vi "EXECUTION_UI.vi"(8 "error in (no error)":errorcluster, 11 "Execution in":refnum<data-value>) -> (0 "error out":errorcluster, 3 "Execution out":refnum<data-value>)   [LabVIEW 2015, in "Execution.lvclass"]
uses:
  Execution.lvclass
  EXECUTION_UI_MSG.ctl
  EXECUTION_CTRL_MSG.ctl
  <vilib>/Utility/miscctls.llb/LVRectTypeDef.ctl
  <vilib>/Utility/miscctls.llb/LVPointTypeDef.ctl
  <vilib>/Utility/miscctls.llb/LVRowAndColumnTypeDef.ctl
  DUT_INFO_TYPEDEF.ctl
  EXECUTION_RESULT_TYPEDEF.ctl
  EXECUTION_STATUS.ctl
  BACKGROUND_CONTROL_MSG_TYPEDEF.ctl
  Step/STEP_STATUS.ctl
  STEP_END_DATA_TYPEDEF.ctl
  <vilib>/Utility/miscctls.llb/LVRowAndColumnUnsignedTypeDef.ctl
  Send UI Message.vi
  Send Control Message.vi
  Project.lvclass
  Step.lvclass
panel:
  out "STOP_FLAG":bool
  out "TEST_TIME":string
  in  "MENU_BTN":bool
  in  "CTRL_BTN":bool
  out "PROGRASS_BAR":u8(slide) scale=0.0..100.0
  out "STATUS":string
  out "SN":string
  out "TEST_TABLE":string[][](table)
  out "Msg":string
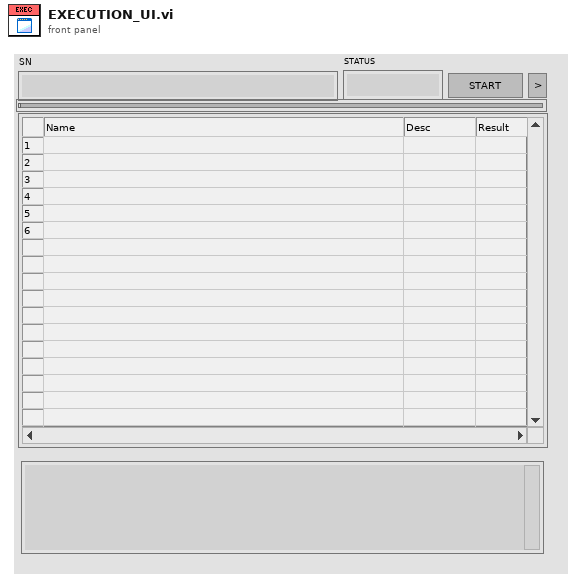
[diagram p1: front panel]
types:
  T1 = typedef "Execution.lvclass/EXECUTION_UI_MSG.ctl" = enum16{"EXECUTION_STATUS", "INIT_UI", "DUT_UPDATE", "BOTTOM_PANEL_UPDATE", "TOP_PANEL_UPDATE", "STEP_START", "STEP_END", "DISPLAY_RESULT", "APPLICATION_END"}
  T2 = typedef "LVRectTypeDef.ctl" = cluster{"Left":i16, "Top":i16, "Right":i16, "Bottom":i16}
  T3 = typedef "LVPointTypeDef.ctl" = cluster{"Horizontal":i16, "Vertical":i16}
  T4 = typedef "LVRowAndColumnTypeDef.ctl" = cluster{"Row":i32, "Column":i32}
  T5 = typedef "Execution.lvclass/DUT_INFO_TYPEDEF.ctl" = cluster{"SN":string, "Model":string, "PartNumber":string, "Revision":string, "Software":string, "Hardware":string}
  T6 = typedef "Execution.lvclass/EXECUTION_RESULT_TYPEDEF.ctl" = enum16{"Unknow", "Terminated", "Passed", "Failed", "Error"}
  T7 = typedef "Execution.lvclass/EXECUTION_STATUS.ctl" = enum16{"Initializing ", "Disable", "Ready", "Running", "Finished"}
  T8 = enum8{"Enabled", "Disabled", "Disabled and Grayed Out"}
  T9 = typedef "Execution.lvclass/BACKGROUND_CONTROL_MSG_TYPEDEF.ctl" = cluster{"Target":string, "Msg":string, "Data":variant}
  T10 = typedef "LVRowAndColumnUnsignedTypeDef.ctl" = cluster{"Row":u32, "Column":u32}
  T11 = typedef "Execution.lvclass/STEP_END_DATA_TYPEDEF.ctl" = cluster{"Index":i32, "Result":T12, "Duration":dbl, "Value":string, "Low Limit":string, "Upper Limit":string}
  T12 = typedef "Step.lvclass/STEP_STATUS.ctl" = enum16{"Skipped", "Done", "Passed", "Failed", "Error"}
  T13 = typedef "Execution.lvclass/EXECUTION_CTRL_MSG.ctl" = enum16{"EXECUTION_START", "EXECUTION_END", "EXECUTION_LOOP", "APPLICATION_STOP"}
  T14 = typedef "Execution.lvclass/EXECUTION_UI_QUEUE_DATA.ctl" = cluster{"Msg":T1, "Data":variant}
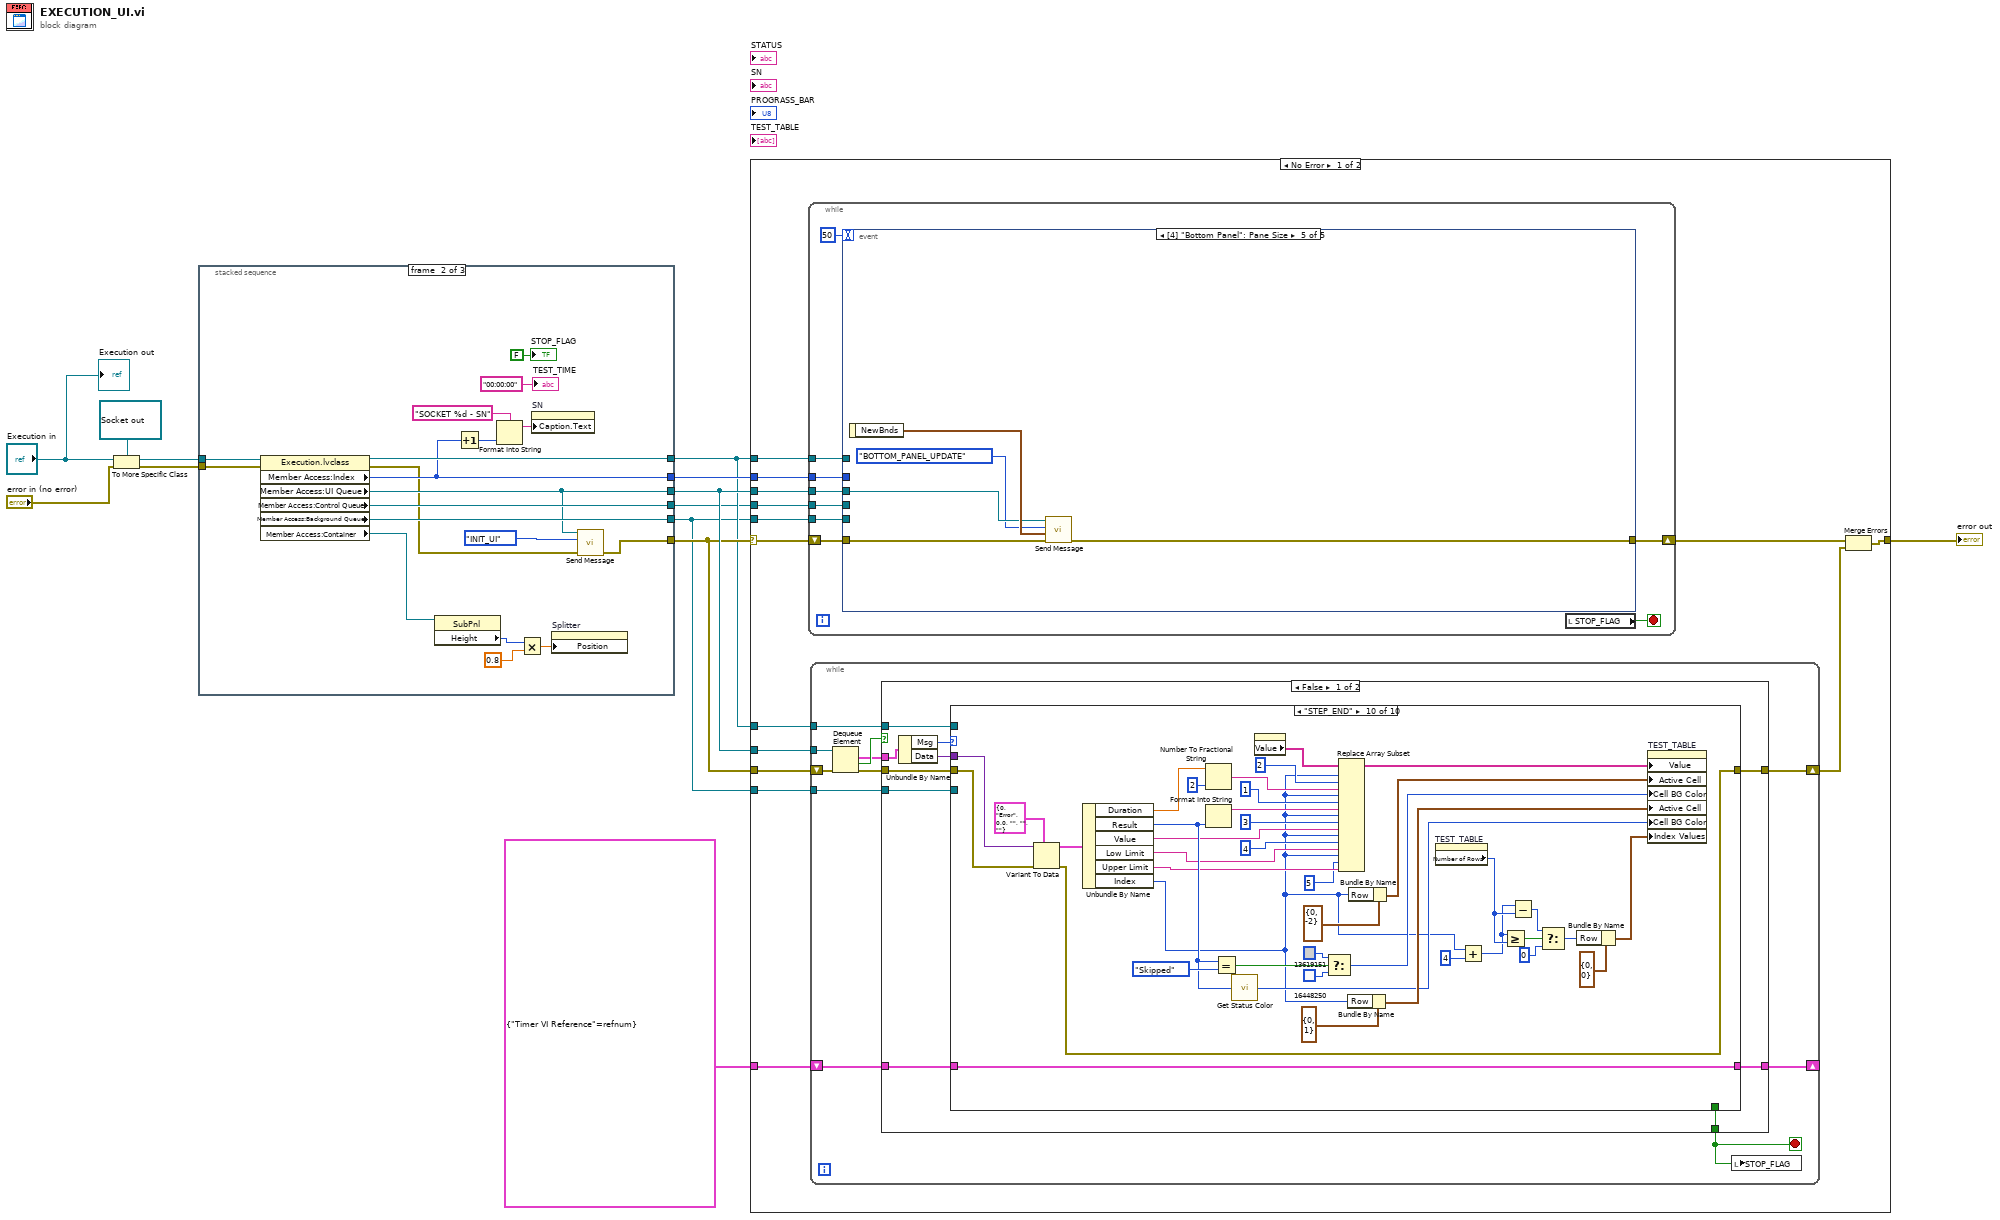
[diagram p0: block diagram]
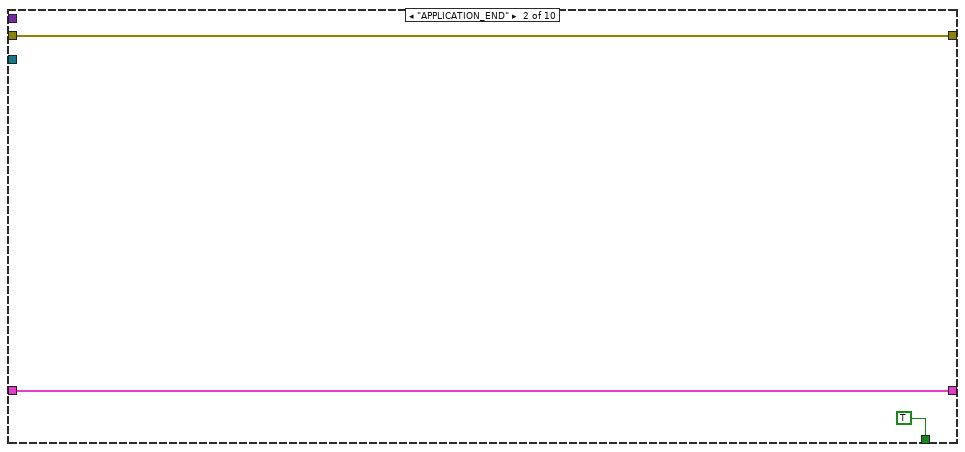
[diagram p5: hidden frame]
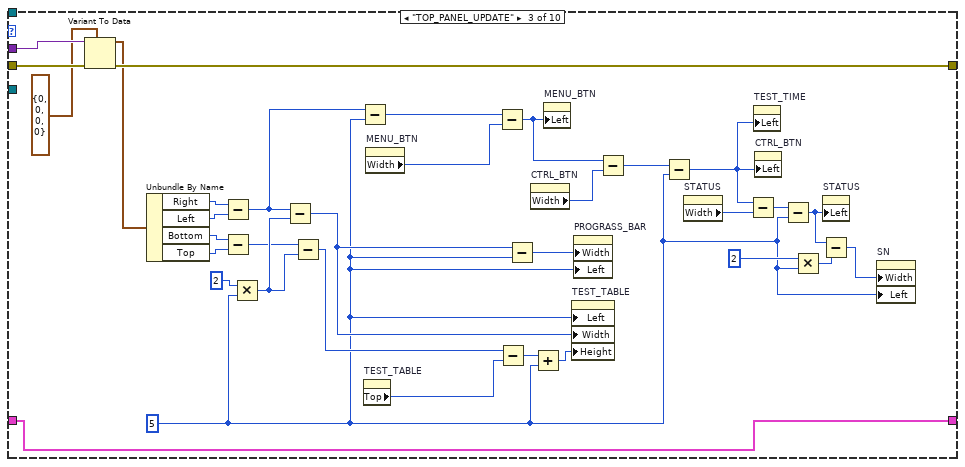
[diagram p6: hidden frame]
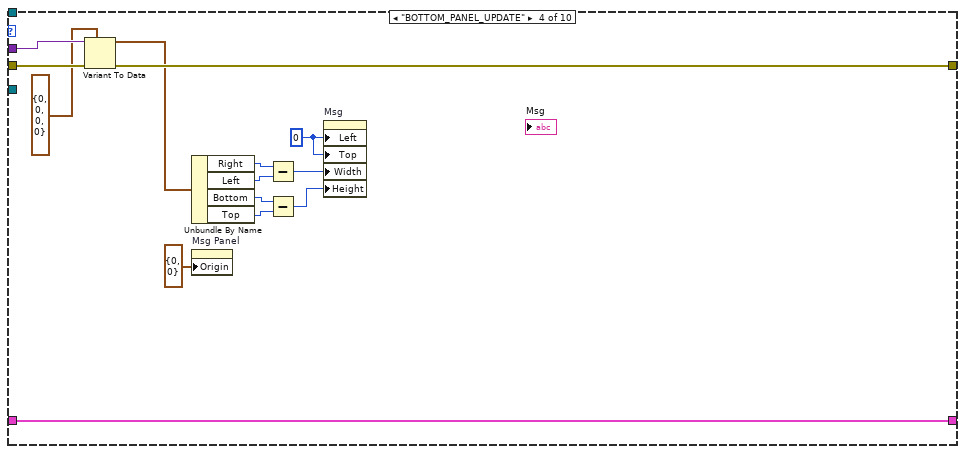
[diagram p7: hidden frame]
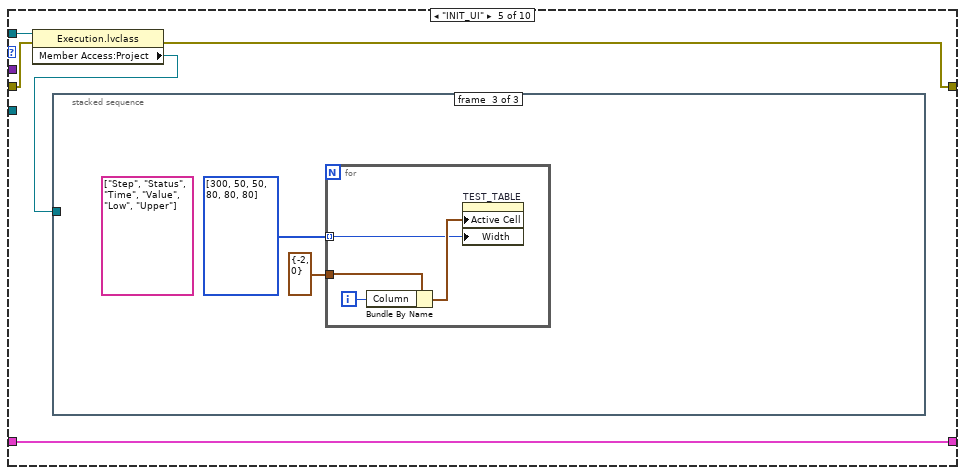
[diagram p8: hidden frame]
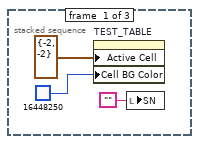
[diagram p9: hidden frame]
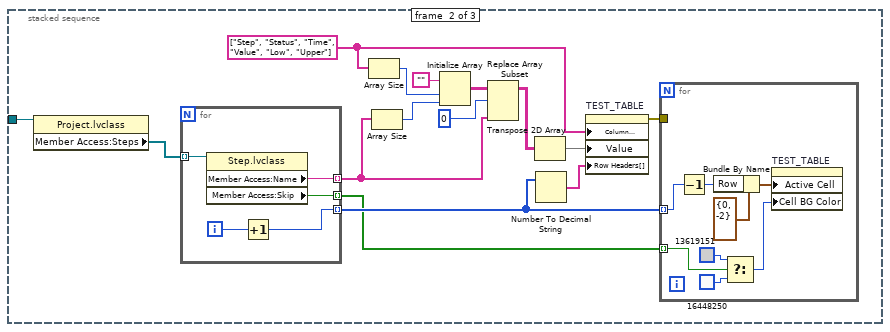
[diagram p10: hidden frame]
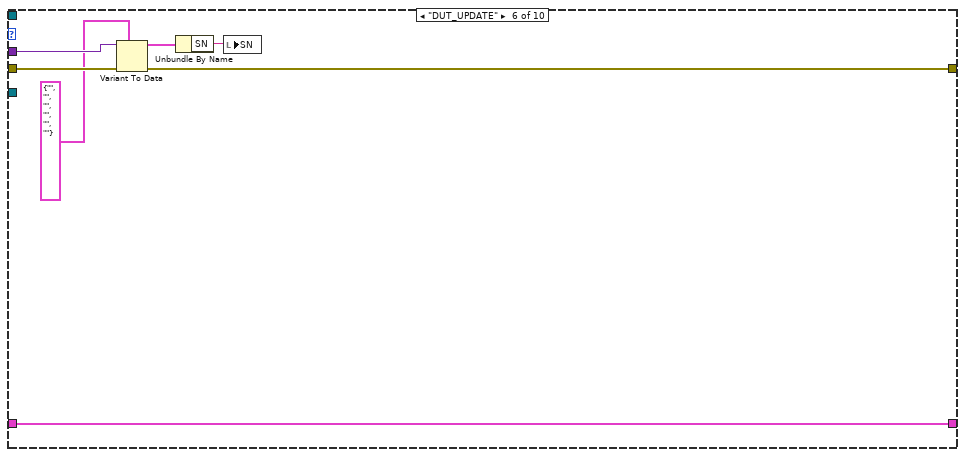
[diagram p11: hidden frame]
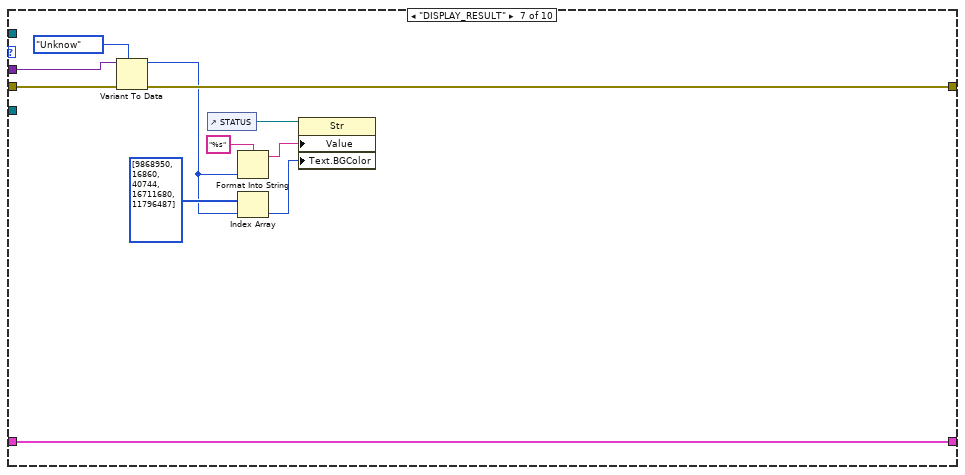
[diagram p12: hidden frame]
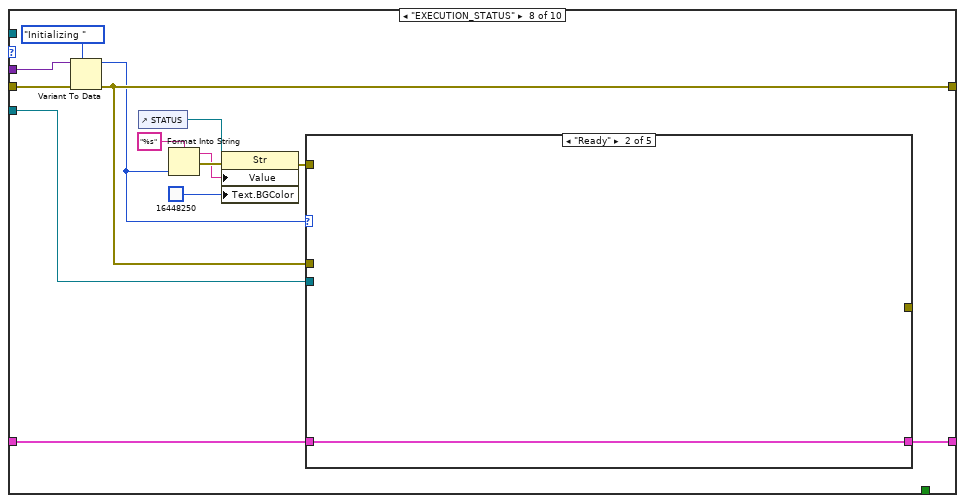
[diagram p13: hidden frame]
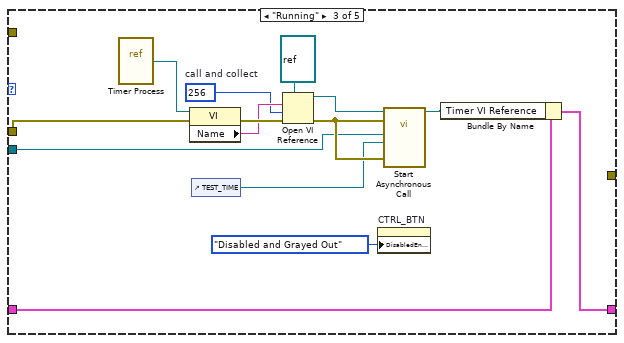
[diagram p15: hidden frame]
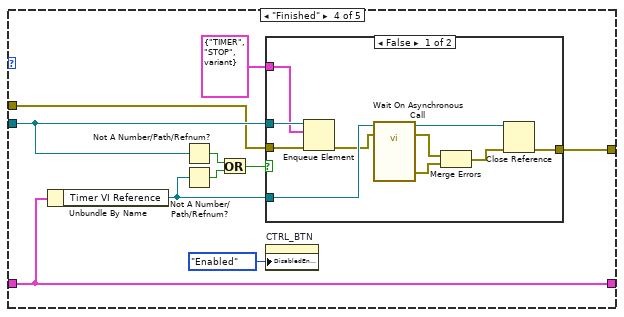
[diagram p16: hidden frame]
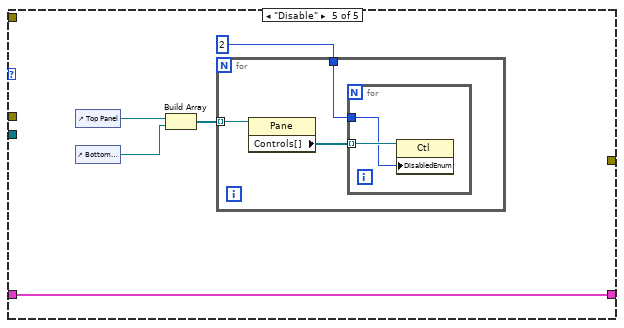
[diagram p18: hidden frame]
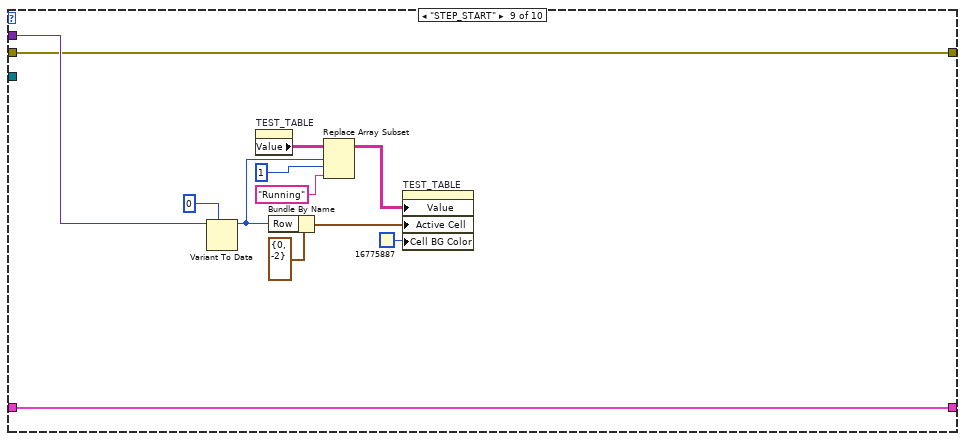
[diagram p19: hidden frame]
diagram:
  n1 = To More Specific Class(target class=refnum<data-value> refnum ("reference out"), reference="Execution in", error in="error in (no error)") -> (specific class reference=w3:refnum<data-value>, error out=w1:errorcluster)
  n2 = stacked-sequence {
    tunnel: [_ w27 _] -> w12
    tunnel: [_ w17 _] -> w11
    tunnel: [_ w14 _] -> w10
    tunnel: [_ w32 _] -> w8
    tunnel: [_ w21 _] -> w7
    tunnel: [_ w20 _] -> w6
    tunnel: w3 -> [_ w19 _]
    tunnel: w1 -> [_ w18 _]
    frame #0 {
    }
    frame #1 {
      n3 = property class="Execution.lvclass"(reference=w19, error in=w18) -> (reference out=w32:refnum<data-value>, error out=w15:errorcluster, "Member Access:Index"=w27:u8, "Member Access:UI Queue"=w17:refnum<queue>, "Member Access:Control Queue"=w20:refnum<queue>, "Member Access:Background Queue"=w21:refnum<queue>, "Member Access:Container"=w22:refnum<vi>)
      n4 = property class="SubPnl"(reference=w22) -> ("Height"=w31:u32)  [unwired: 1 in, 2 out]
      n5 = Increment(x=w27) -> (x+1=w25:u8)
      n6 = Format Into String(format string="SOCKET %d - SN", w25) -> (resulting string=w24:string)  [unwired: 2 in, 1 out]
      n7 = Multiply(x=w31, y=0.8) -> (x*y=w30:dbl)
      n8 = property on="SN" class="Str"("Caption.Text"=w24) -> ()  [unwired: 2 in, 2 out]
      n9 = property on="Splitter" class="Splitter"("Position"=w30) -> ()  [unwired: 2 in, 2 out]
      n10 = call-poly "Send Message.vi"("error in (no error)"=w15, "Msg"=EXECUTION_UI_MSG."INIT_UI", "UI Queue"=w17) -> ("error out"=w14:errorcluster)  [unwired: 8 in]
      "TEST_TIME" <- "00:00:00" ("String")
      "STOP_FLAG" <- FALSE ("STOP_FLAG")
    }
    frame #2 {
    }
  }
  n11 = case shown="No Error" w10 {
    selector: w10 -> [w46 w319]
    tunnel: [w38 w319] -> w13
    tunnel: w11 -> [w45 _]
    tunnel: w12 -> [w44 _]
    tunnel: w8 -> [w43 _]
    tunnel: w11 -> [w42 _]
    tunnel: w10 -> [w41 _]
    tunnel: w7 -> [w37 _]
    tunnel: cluster{"Timer VI Reference":refnum<vi>} {"Timer VI Reference"=refnum} -> [w36 _]
    tunnel: w8 -> [w35 _]
    tunnel: w7 -> [w34 _]
    tunnel: w6 -> [w33 _]
    frame No Error {
      n12 = while {
        tunnel: w45 -> [w300]
        tunnel: w44 -> [w299]
        shift-right: [w302] -> w40
        shift-left: w46 -> [w303]
        tunnel: w43 -> [w298]
        tunnel: w34 -> [w296]
        tunnel: w33 -> [w295]
        stop <- w297 stop-if-true
        n13 = event shown="[4] \"Bottom Panel\": Pane Size" {
          selector: _ -> [_ _ _ _ _]
          dyn-events: _ -> [_ _ _ _ _]
          timeout: 50 -> [_ _ _ _ _]
          tunnel: w303 -> [w304 w308 _ w313 w315]
          tunnel: [w304 w307 _ w309 w314] -> w302
          tunnel: w300 -> [_ _ _ w312 w317]
          tunnel: w299 -> [_ _ _ _ _]
          tunnel: w298 -> [_ _ _ _ _]
          tunnel: w296 -> [_ _ _ _ _]
          tunnel: w295 -> [_ w306 _ _ _]
          event Timeout {
            n14 = event-data() -> ()  [unwired: 1 in, 3 out]
          }
          event "CTRL_BTN": Value Change {
            n15 = event-data() -> ()  [unwired: 1 in, 6 out]
            n16 = call-poly "Send Message.vi"("error in (no error)"=w308, "Msg"=EXECUTION_CTRL_MSG."EXECUTION_START", "Control Queue"=w306) -> ("error out"=w307:errorcluster)  [unwired: 8 in]
          }
          event "MENU_BTN": Value Change {
            n17 = event-data() -> ()  [unwired: 1 in, 6 out]
          }
          event Pane Size {
            n18 = event-data() -> ("NewBnds"=w310:T2)  [unwired: 1 in]
            n19 = call-poly "Send Message.vi"("error in (no error)"=w313, "Data"=w310, "Msg"=EXECUTION_UI_MSG."TOP_PANEL_UPDATE", "UI Queue"=w312) -> ("error out"=w309:errorcluster)  [unwired: 7 in]
          }
          event Pane Size {
            n20 = event-data() -> ("NewBnds"=w318:T2)  [unwired: 1 in]
            n21 = call-poly "Send Message.vi"("error in (no error)"=w315, "Data"=w318, "Msg"=EXECUTION_UI_MSG."BOTTOM_PANEL_UPDATE", "UI Queue"=w317) -> ("error out"=w314:errorcluster)  [unwired: 7 in]
          }
        }
        n22 = local read "STOP_FLAG"() -> (w297:bool)
      }
      n23 = while {
        tunnel: w42 -> [w57]
        shift-right: [w52] -> w39
        shift-left: w41 -> [w56]
        tunnel: w37 -> [w49]
        shift-right: [w48] -> _
        shift-left: w36 -> [w50]
        tunnel: w35 -> [w47]
        stop <- w51 stop-if-true
        n24 = Dequeue Element(queue=w57, error in (no error)=w56) -> (element=w54:T14, timed out?=w55:bool, error out=w53:errorcluster)  [unwired: 1 in, 1 out]
        n25 = case shown="False" w55 {
          tunnel: w53 -> [w64 w294]
          tunnel: w54 -> [w65 _]
          tunnel: [w67 w294] -> w52
          tunnel: [w66 _] -> w51
          tunnel: w50 -> [w61 w293]
          tunnel: w49 -> [w60 _]
          tunnel: [w59 w293] -> w48
          tunnel: w47 -> [w58 _]
          frame False {
            n26 = Unbundle By Name(w65) -> ("Msg"=w63:T1, "Data"=w62:variant)
            n27 = case shown="\"STEP_END\"" w63 {
              tunnel: w64 -> [w69 w72 w78 w118 w121 w167 w178 w193 w247 w270]
              tunnel: [w69 w72 w77 w117 w120 w163 w177 w189 w247 w269] -> w67
              tunnel: [_ TRUE _ _ _ _ _ _ _ _] -> w66
              tunnel: w62 -> [_ _ w79 w119 _ w168 w179 w192 w249 w291]
              tunnel: w61 -> [w68 w70 w73 w106 w122 w162 w176 w190 w251 w292]
              tunnel: w60 -> [_ _ _ _ _ _ _ w188 _ _]
              tunnel: [w68 w70 w73 w106 w122 w162 w176 w187 w251 w292] -> w59
              tunnel: w58 -> [_ _ _ _ w124 _ _ _ _ _]
              frame Default {
              }
              frame "APPLICATION_END" {
              }
              frame "TOP_PANEL_UPDATE" {
                w74 = 5
                n28 = Variant To Data(error in=w78, type=T2 {"Left"=0, "Top"=0, "Right"=0, "Bottom"=0} ("NewBnds"), Variant=w79) -> (data=w75:T2, error out=w77:errorcluster)
                n29 = Unbundle By Name(w75) -> ("Right"=w81:i16, "Left"=w80:i16, "Bottom"=w83:i16, "Top"=w82:i16)
                n30 = Subtract(x=w81, y=w80) -> (x-y=w87:i16)
                n31 = Subtract(x=w83, y=w82) -> (x-y=w84:i16)
                n32 = Multiply(x=2, y=w74) -> (x*y=w86:i32)
                n33 = Subtract(x=w87, y=w86) -> (x-y=w102:i32)
                n34 = Subtract(x=w84, y=w86) -> (x-y=w98:i32)
                n35 = Subtract(x=w87, y=w74) -> (x-y=w88:i32)
                n36 = property on="TEST_TABLE" class="Tbl (strict)"() -> ("Top"=w99:i32)  [unwired: 2 in, 2 out]
                n37 = property on="MENU_BTN" class="Bool"() -> ("Width"=w89:u32)  [unwired: 2 in, 2 out]
                n38 = Subtract(x=w88, y=w89) -> (x-y=w90:u32)
                n39 = Subtract(x=w98, y=w99) -> (x-y=w100:i32)
                n40 = Subtract(x=w102, y=w74) -> (x-y=w103:i32)
                n41 = property on="CTRL_BTN" class="Bool"() -> ("Width"=w91:u32)  [unwired: 2 in, 2 out]
                n42 = Add(x=w100, y=w74) -> (x+y=w101:i32)
                n43 = property on="MENU_BTN" class="Bool"("Left"=w90) -> ()  [unwired: 2 in, 2 out]
                n44 = property on="TEST_TABLE" class="Tbl (strict)"("Left"=w74, "Width"=w102, "Height"=w101) -> ()  [unwired: 2 in, 2 out]
                n45 = property on="PROGRASS_BAR" class="Slide (strict)"("Width"=w103, "Left"=w74) -> ()  [unwired: 2 in, 2 out]
                n46 = Subtract(x=w90, y=w91) -> (x-y=w92:u32)
                n47 = Subtract(x=w92, y=w74) -> (x-y=w104:u32)
                n48 = property on="STATUS" class="Str"() -> ("Width"=w93:u32)  [unwired: 2 in, 2 out]
                n49 = Subtract(x=w104, y=w93) -> (x-y=w94:u32)
                n50 = property on="TEST_TIME" class="Str"("Left"=w104) -> ()  [unwired: 2 in, 2 out]
                n51 = property on="CTRL_BTN" class="Bool"("Left"=w104) -> ()  [unwired: 2 in, 2 out]
                n52 = Subtract(x=w94, y=w74) -> (x-y=w105:u32)
                n53 = Multiply(x=2, y=w74) -> (x*y=w95:i32)
                n54 = Subtract(x=w105, y=w95) -> (x-y=w97:u32)
                n55 = property on="STATUS" class="Str"("Left"=w105) -> ()  [unwired: 2 in, 2 out]
                n56 = property on="SN" class="Str"("Width"=w97, "Left"=w74) -> ()  [unwired: 2 in, 2 out]
              }
              frame "BOTTOM_PANEL_UPDATE" {
                w108 = 0 ("Position:Left")
                n57 = Variant To Data(error in=w118, type=T2 {"Left"=0, "Top"=0, "Right"=0, "Bottom"=0} ("NewBnds"), Variant=w119) -> (data=w107:T2, error out=w117:errorcluster)
                n58 = Unbundle By Name(w107) -> ("Right"=w110:i16, "Left"=w109:i16, "Bottom"=w112:i16, "Top"=w111:i16)
                n59 = property on="Msg Panel" class="Pane"("Origin"=T3 {"Horizontal"=0, "Vertical"=0}) -> ()  [unwired: 2 in, 2 out]
                n60 = Subtract(x=w110, y=w109) -> (x-y=w113:i16)
                n61 = Subtract(x=w112, y=w111) -> (x-y=w114:i16)
                n62 = property on="Msg" class="Str"("Left"=w108, "Top"=w108, "Width"=w113, "Height"=w114) -> ()  [unwired: 2 in, 2 out]
              }
              frame "INIT_UI" {
                n63 = property class="Execution.lvclass"(reference=w124, error in=w121) -> (error out=w120:errorcluster, "Member Access:Project"=w123:refnum<class "Project.lvclass">)  [unwired: 1 out]
                n64 = stacked-sequence {
                  tunnel: w123 -> [_ w142 _]
                  frame #0 {
                    n65 = property on="TEST_TABLE" class="Tbl (strict)"("Active Cell"=T4 {"Row"=-2, "Column"=-2} ("Active Cell:Active Cell"), "Cell BG Color"=u32 16448250) -> ()  [unwired: 2 in, 2 out]
                    n66 = local write "SN"("") -> ()
                  }
                  frame #1 {
                    w134 = string[] ["Step", "Status", "Time", "Value", "Low", "Upper"] ("Column Header Strings[]")
                    n67 = property class="Project.lvclass"(reference=w142) -> ("Member Access:Steps"=w141:refnum<class "Step.lvclass">[])  [unwired: 1 in, 2 out]
                    n68 = for {
                      tunnel: w141 -> [w155] mode=indexing
                      tunnel: [w154] -> w137 mode=indexing
                      tunnel: [w153] -> w129 mode=indexing
                      tunnel: [w151] -> w138 mode=indexing
                      i -> [w152]
                      n69 = property class="Step.lvclass"(reference=w155) -> ("Member Access:Name"=w153:string, "Member Access:Skip"=w154:bool)  [unwired: 1 in, 2 out]
                      n70 = Increment(x=w152) -> (x+1=w151:i32)
                    }
                    n71 = Array Size(array=w134) -> (size(s)=w133:i32)
                    n72 = Array Size(array=w129) -> (size(s)=w132:i32)
                    n73 = Initialize Array("", w133, w132) -> (w131:string[][])
                    n74 = Replace Array Subset(array=w131, new element=w129, index (row)=0) -> (w128:string[][])  [unwired: 1 in]
                    n75 = Transpose 2D Array(2D array=w128) -> (transposed array=w136:string[][])
                    n76 = Number To Decimal String(number=w138) -> (decimal integer string=w140:string[])  [unwired: 1 in]
                    n77 = property on="TEST_TABLE" class="Tbl (strict)"("Column Headers[]"=w134, "Value"=w136, "Row Headers[]"=w140) -> (error out=w139:errorcluster)  [unwired: 2 in, 1 out]
                    n78 = for {
                      tunnel: w139 -> [_]
                      tunnel: w138 -> [w144] mode=indexing
                      tunnel: w137 -> [w147] mode=indexing
                      n79 = Decrement(x=w144) -> (x-1=w143:i32)
                      n80 = Bundle By Name(cluster=T4 {"Row"=0, "Column"=-2} ("Active Cell:Active Cell"), "Row"=w143) -> (w149:T4)
                      n81 = Select(t=u32 13619151, s=w147, f=u32 16448250) -> (s? t:f=w146:u32)
                      n82 = property on="TEST_TABLE" class="Tbl (strict)"("Active Cell"=w149, "Cell BG Color"=w146) -> ()  [unwired: 2 in, 2 out]
                    }
                  }
                  frame #2 {
                    (unwired) string[] ["Step", "Status", "Time", "Value", "Low", "Upper"] ("Column Header Strings[]")
                    n83 = for {
                      tunnel: T4 {"Row"=-2, "Column"=0} ("Active Cell:Active Cell") -> [w161]
                      tunnel: i32[] [300, 50, 50, 80, 80, 80] -> [w158] mode=indexing
                      i -> [w160]
                      n84 = Bundle By Name(cluster=w161, "Column"=w160) -> (w159:T4)
                      n85 = property on="TEST_TABLE" class="Tbl (strict)"("Active Cell"=w159, "Width"=w158) -> ()  [unwired: 2 in, 2 out]
                    }
                  }
                }
              }
              frame "DUT_UPDATE" {
                n86 = Variant To Data(error in=w167, type=T5 {"SN"="", "Model"="", "PartNumber"="", "Revision"="", "Software"="", "Hardware"=""} ("DUT INFO"), Variant=w168) -> (data=w165:T5, error out=w163:errorcluster)
                n87 = Unbundle By Name(w165) -> ("SN"=w164:string)
                n88 = local write "SN"(w164) -> ()
              }
              frame "DISPLAY_RESULT" {
                n89 = Variant To Data(error in=w178, type=EXECUTION_RESULT_TYPEDEF."Unknow" ("Execution Result"), Variant=w179) -> (data=w170:T6, error out=w177:errorcluster)
                n90 = control-ref of="STATUS"() -> (w173:refnum<vi>)
                n91 = Format Into String(format string="%s", w170) -> (resulting string=w172:string)  [unwired: 2 in, 1 out]
                n92 = Index Array(array=u32[] [9868950, 16860, 40744, 16711680, 11796487], index=w170) -> (element=w169:u32)
                n93 = property class="Str"(reference=w173, "Value"=w172, "Text.BGColor"=w169) -> ()  [unwired: 1 in, 2 out]
              }
              frame "EXECUTION_STATUS" {
                n94 = Variant To Data(error in=w193, type=EXECUTION_STATUS."Initializing " ("Status"), Variant=w192) -> (data=w185:T7, error out=w189:errorcluster)
                n95 = control-ref of="STATUS"() -> (w183:refnum<vi>)
                n96 = Format Into String(format string="%s", w185) -> (resulting string=w182:string, error out=w184:errorcluster)  [unwired: 2 in]
                n97 = property class="Str"(reference=w183, error in=w184, "Value"=w182, "Text.BGColor"=u32 16448250) -> (error out=w180:errorcluster)  [unwired: 1 out]
                n98 = case shown="\"Ready\"" w185 {
                  tunnel: w190 -> [w194 w195 w200 w211 w230]
                  tunnel: w189 -> [_ _ w202 w214 _]
                  tunnel: w188 -> [_ _ w201 w216 _]
                  tunnel: [w194 w195 w198 w211 w230] -> w187
                  tunnel: [_ _ _ w212 _] -> _
                  tunnel: w180 -> [_ _ _ _ _]
                  frame "Initializing ", Default {
                  }
                  frame "Ready" {
                  }
                  frame "Running" {
                    w204 = 256  # call and collect
                    n99 = vi-ref "Timer Process.vi"() -> (w206:refnum<vi>)
                    n100 = property class="VI"(reference=w206, error in=w202) -> (error out=w208:errorcluster, "Name"=w207:string)  [unwired: 1 out]
                    n101 = control-ref of="TEST_TIME"() -> (w197:refnum<vi>)
                    n102 = Open VI Reference(type specifier VI Refnum (for type only)=refnum<vi> refnum ("VI Refnum"), vi path=w207, options=w204, error in (no error)=w208) -> (vi reference=w205:refnum<vi>, error out=w209:errorcluster)  [unwired: 2 in]
                    n103 = property on="CTRL_BTN" class="Bool"("DisabledEnum"=T8."Disabled and Grayed Out" ("Disabled")) -> ()  [unwired: 2 in, 2 out]
                    n104 = call-by-ref "Start Asynchronous Call"(reference=w205, error in=w209, 8:"error in (no error)"=w209, "Timer Display Refnum"=w197, "Background Control Queue"=w201) -> (reference out=w199:refnum<vi>)  [unwired: 8 in, 2 out]
                    n105 = Bundle By Name(cluster=w200, "Timer VI Reference"=w199) -> (w198:cluster{"Timer VI Reference":refnum<vi>})
                  }
                  frame "Finished" {
                    n106 = Unbundle By Name(w211) -> ("Timer VI Reference"=w213:refnum<vi>)
                    n107 = Not A Number/Path/Refnum?(number/path/refnum=w216) -> (NaN/Path/Refnum?=w218:bool)
                    n108 = Not A Number/Path/Refnum?(number/path/refnum=w213) -> (NaN/Path/Refnum?=w219:bool)
                    n109 = Or(x=w218, y=w219) -> (x .or. y?=w217:bool)
                    n110 = case shown="False" w217 {
                      tunnel: w216 -> [w229 _]
                      tunnel: T9 {"Target"="TIMER", "Msg"="STOP", "Data"=variant} ("element") -> [w228 _]
                      tunnel: w214 -> [w227 _]
                      tunnel: w213 -> [w222 _]
                      tunnel: [w220 _] -> w212
                      frame False {
                        n111 = Enqueue Element(queue=w229, element=w228, error in (no error)=w227) -> (error out=w221:errorcluster)  [unwired: 1 in, 2 out]
                        n112 = call-by-ref "Wait On Asynchronous Call"(reference=w222, error in=w221) -> (reference out=w223:refnum<vi>, error out=w224:errorcluster, 0:"error out"=w225:errorcluster)  [unwired: 11 in]
                        n113 = Merge Errors(w224, w225) -> (w226:errorcluster)
                        n114 = Close Reference(reference=w223, error in (no error)=w226) -> (error out=w220:errorcluster)
                      }
                      frame True {
                      }
                    }
                    n115 = property on="CTRL_BTN" class="Bool"("DisabledEnum"=T8."Enabled" ("Disabled")) -> ()  [unwired: 2 in, 2 out]
                  }
                  frame "Disable" {
                    n116 = control-ref of="Top Panel"() -> (w234:refnum<vi>)
                    n117 = control-ref of="Bottom Panel"() -> (w233:refnum<vi>)
                    n118 = Build Array(w234, w233) -> (w232:refnum<vi>[])
                    n119 = for {
                      tunnel: u8 2 ("f") -> [w237]
                      tunnel: w232 -> [w236] mode=indexing
                      n120 = property class="Pane"(reference=w236) -> ("Controls[]"=w235:refnum<vi>[])  [unwired: 1 in, 2 out]
                      n121 = for {
                        tunnel: w235 -> [w239] mode=indexing
                        tunnel: w237 -> [w238]
                        n122 = property class="Ctl"(reference=w239, "DisabledEnum"=w238) -> ()  [unwired: 1 in, 2 out]
                      }
                    }
                  }
                }
              }
              frame "STEP_START" {
                n123 = Variant To Data(type=u32 0, Variant=w249) -> (data=w242:u32)  [unwired: 1 in, 1 out]
                n124 = property on="TEST_TABLE" class="Tbl (strict)"() -> ("Value"=w244:string[][])  [unwired: 2 in, 2 out]
                n125 = Bundle By Name(cluster=T4 {"Row"=0, "Column"=-2} ("Active Cell:Active Cell"), "Row"=w242) -> (w246:T4)
                n126 = Replace Array Subset(array=w244, new element="Running", index (row)=w242, index (col)=1) -> (w240:string[][])
                n127 = property on="TEST_TABLE" class="Tbl (strict)"("Value"=w240, "Active Cell"=w246, "Cell BG Color"=u32 16775887) -> ()  [unwired: 2 in, 2 out]
              }
              frame "STEP_END" {
                n128 = Variant To Data(error in=w270, type=T11 {"Index"=0, "Result"=enum."Error", "Duration"=0.0, "Value"="", "Low Limit"="", "Upper Limit"=""}, Variant=w291) -> (data=w288:T11, error out=w269:errorcluster)
                n129 = Unbundle By Name(w288) -> ("Duration"=w273:dbl, "Result"=w280:T12, "Value"=w267:string, "Low Limit"=w265:string, "Upper Limit"=w264:string, "Index"=w254:i32)
                n130 = Number To Fractional String(number=w273, precision (6)=i16 2) -> (F-format string=w272:string)  [unwired: 2 in]
                n131 = Format Into String(w280) -> (resulting string=w275:string)  [unwired: 3 in, 1 out]
                n132 = Equal?(x=w280, y=STEP_STATUS."Skipped") -> (x = y?=w281:bool)
                n133 = call "Get Status Color.vi"("Status"=w280) -> ("Color"=w277:u32)
                n134 = property on="TEST_TABLE" class="Tbl (strict)"() -> ("Value"=w287:string[][])  [unwired: 2 in, 2 out]
                n135 = Select(t=u32 13619151, s=w281, f=u32 16448250) -> (s? t:f=w283:u32)
                n136 = Replace Array Subset(array=w287, new element #1=w272, index (row) #1=w254, index (col) #1=2, new element #2=w275, index (row) #2=w254, index (col) #2=1, new element #3=w267, index (row) #3=w254, index (col) #3=3, new element #4=w265, index (row) #4=w254, index (col) #4=4, new element #5=w264, index (row) #5=w254, index (col) #5=5) -> (w259:string[][])
                n137 = Bundle By Name(cluster=T4 {"Row"=0, "Column"=1} ("Active Cell:Active Cell"), "Row"=w254) -> (w278:T4)
                n138 = Bundle By Name(cluster=T4 {"Row"=0, "Column"=-2} ("Active Cell:Active Cell"), "Row"=w254) -> (w289:T4)
                n139 = property on="TEST_TABLE" class="Tbl (strict)"() -> ("Number of Rows"=w255:u32)  [unwired: 2 in, 2 out]
                n140 = Add(x=w254, y=4) -> (x+y=w252:i32)
                n141 = Greater Or Equal?(x=w252, y=w255) -> (x >= y?=w257:bool)
                n142 = Subtract(x=w252, y=w255) -> (x-y=w256:u32)
                n143 = Select(t=w256, s=w257, f=u32 0) -> (s? t:f=w262:u32)
                n144 = Bundle By Name(cluster=T10 {"Row"=0, "Column"=0} ("Index Values"), "Row"=w262) -> (w258:T10)
                n145 = property on="TEST_TABLE" class="Tbl (strict)"("Value"=w259, "Active Cell"=w289, "Cell BG Color"=w283, "Active Cell"=w278, "Cell BG Color"=w277, "Index Values"=w258) -> ()  [unwired: 2 in, 2 out]
              }
            }
          }
          frame True {
          }
        }
        n146 = local write "STOP_FLAG"(w51) -> ()
      }
      n147 = Merge Errors(w40, w39) -> (w38:errorcluster)
    }
    frame Error {
    }
  }
  "error out" <- w13
  "Execution out" <- "Execution in"
